vi "Write Data Xfer.vi"(8 "Error In":errorcluster, 9 "Time Stamp":dbl format="%^<%H:%M:%S%4u\n%x>T", 10 "Data Value":dbl, 11 "Device Name":string) -> (0 "Error Out":errorcluster)   [LabVIEW 2014]
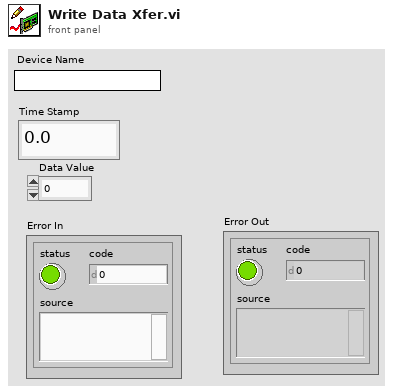
[diagram p1: front panel]
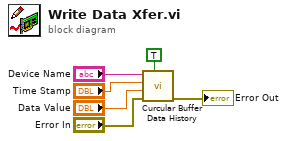
[diagram p0: block diagram]
diagram:
  n1 = call "Curcular Buffer Data History.vi"("write (F)"=TRUE, "Error In"="Error In", "Data Value"="Data Value", "Time Stamp"="Time Stamp", "Device Name"="Device Name") -> ("Error Out"=→"Error Out":errorcluster)  [unwired: 3 in, 3 out]
